vi "S2C_FORNAX_Proc_ReadSettings.vi"(8 "Error In":errorcluster) -> (0 "Error Out":errorcluster)   [LabVIEW 2015]
doc: "Reads the data contained within the Fornax Commands file and loads the data into the Fornax global variables."
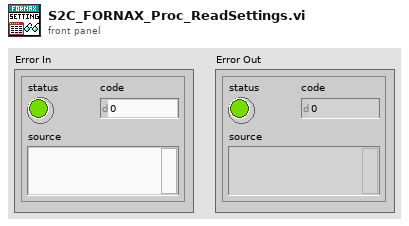
[diagram p1: front panel]
types:
  T1 = enum32{"Bad", "Idle", "Run top level", "Running"}
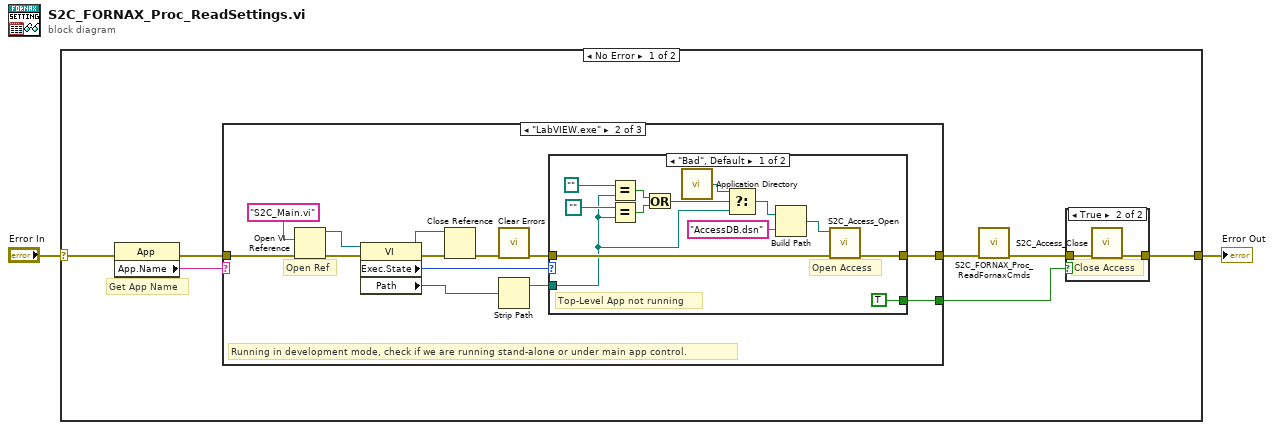
[diagram p0: block diagram]
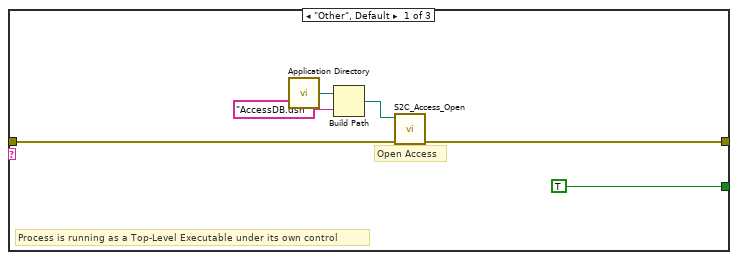
[diagram p2: hidden frame]
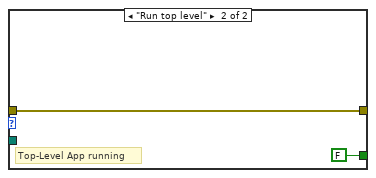
[diagram p3: hidden frame]
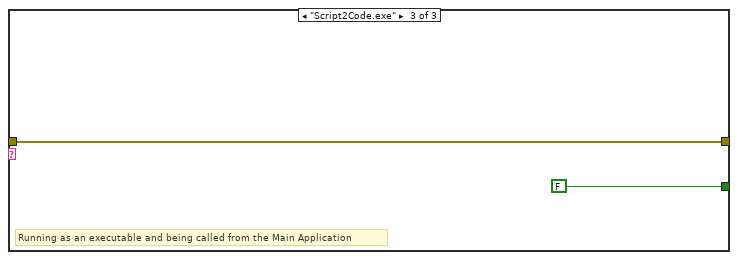
[diagram p4: hidden frame]
diagram:
  n1 = case shown="No Error" "Error In" {
    selector: "Error In" -> [w6 w49]
    tunnel: [w9 w49] -> w1
    frame No Error {
      # "Get App Name"
      n2 = property class="App"(error in=w6) -> (error out=w7:errorcluster, "App.Name"=w8:string)  [unwired: 1 in, 1 out]
      n3 = case shown="\"LabVIEW.exe\"" w8 {
        tunnel: w7 -> [w13 w26 w44]
        tunnel: [w11 w23 w44] -> w4
        tunnel: [TRUE ("Exit?") w22 FALSE ("Exit?")] -> w5
        frame "Other", Default {
          # "Open Access"
          # "Process is running as a Top-Level Executable under its own control"
          n4 = call <vilib>:"Application Directory.vi"() -> ("Application Directory"=w14:path)
          n5 = Build Path(base path=w14, name or relative path="AccessDB.dsn") -> (appended path=w12:path)
          n6 = call "S2C_Access_Open.vi"("Error In"=w13, "DSN_Path"=w12) -> ("Error Out"=w11:errorcluster)  [unwired: 8 in, 1 out]
        }
        frame "LabVIEW.exe" {
          # "Running in development mode, check if we are running stand-alone or under main app control."
          # "Open Ref"
          n7 = Open VI Reference(vi path="S2C_Main.vi" ("element"), error in (no error)=w26) -> (vi reference=w27:refnum<vi>, error out=w28:errorcluster)  [unwired: 4 in]
          n8 = property class="VI"(reference=w27, error in=w28) -> (reference out=w20:refnum<vi>, error out=w21:errorcluster, "Exec.State"=w24:T1, "Path"=w17:path)
          n9 = Close Reference(reference=w20, error in (no error)=w21) -> (error out=w19:errorcluster)
          n10 = call <vilib>:"Clear Errors.vi"("error in (no error)"=w19) -> ("error out"=w18:errorcluster)  [unwired: 5 in, 1 out]
          n11 = Strip Path(path=w17) -> (stripped path=w16:path)  [unwired: 1 out]
          n12 = case shown="\"Bad\", Default" w24 {
            tunnel: [w37 w43] -> w23
            tunnel: [TRUE FALSE] -> w22
            tunnel: w18 -> [w38 w43]
            tunnel: w16 -> [w32 _]
            frame "Bad", Default {
              # "Open Access"
              # "Top-Level App not running"
              n13 = Equal?(x=path "", y=w32) -> (x = y?=w31:bool)
              n14 = Equal?(x=path "", y=w32) -> (x = y?=w30:bool)
              n15 = Or(x=w31, y=w30) -> (x .or. y?=w29:bool)
              n16 = call <vilib>:"Application Directory.vi"() -> ("Application Directory"=w35:path)
              n17 = Select(t=w35, s=w29, f=w32) -> (s? t:f=w34:path)
              n18 = Build Path(base path=w34, name or relative path="AccessDB.dsn") -> (appended path=w39:path)
              n19 = call "S2C_Access_Open.vi"("Error In"=w38, "DSN_Path"=w39) -> ("Error Out"=w37:errorcluster)  [unwired: 8 in, 1 out]
            }
            frame "Run top level" {
              # "Top-Level App running"
            }
          }
        }
        frame "Script2Code.exe" {
          # "Running as an executable and being called from the Main Application"
        }
      }
      n20 = call "S2C_FORNAX_Proc_ReadFornaxCmds.vi"("Error In"=w4) -> ("Error Out"=w3:errorcluster)  [unwired: 10 in]
      n21 = case shown="True" w5 {
        tunnel: w3 -> [w46 w48]
        tunnel: [w46 w47] -> w9
        frame False {
        }
        frame True {
          # "Close Access"
          n22 = call "S2C_Access_Close.vi"("Error In"=w48) -> ("Error Out"=w47:errorcluster)  [unwired: 10 in]
        }
      }
    }
    frame Error {
    }
  }
  "Error Out" <- w1
